vi "write wf.vi"() -> ()   [LabVIEW 2013]
uses:
  <vilib>/addons/database/Connection.llb/DB Tools Open Connec (Path).vi
  <vilib>/measure/NI_MABase.lvlib
  <vilib>/addons/database/NI_Database_API.lvlib
panel:
  out "error out":errorcluster
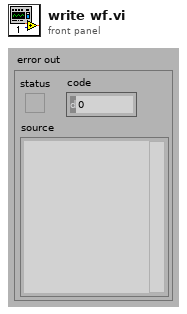
[diagram p1: front panel]
types:
  T1 = enum16{"Sine Wave", "Triangle Wave", "Square Wave", "Sawtooth Wave"}
  T2 = typedef "NI_Database_API.lvlib/Conn ObjectReference.ctl" = refnum<k1>
  T3 = cluster{"table":string, "signal out":waveform(dbl)}
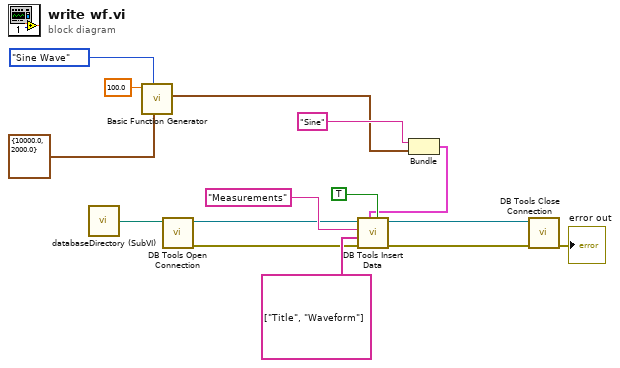
[diagram p0: block diagram]
diagram:
  n1 = call "databaseDirectory (SubVI).vi"() -> ("Application Directory"=w6:path)  [unwired: 1 in]
  n2 = call <vilib>:"Basic Function Generator.vi"("sampling info"=cluster{"Fs":dbl, "#s":dbl} {"Fs"=10000.0, "#s"=2000.0}, "signal type"=T1."Sine Wave", "frequency"=100.0) -> ("signal out"=w1:waveform(dbl))  [unwired: 6 in, 2 out]
  n3 = call-poly <vilib>:"DB Tools Open Connection.vi"("connection information"=w6) -> ("error out"=w5:errorcluster, "connection reference"=w4:T2)  [unwired: 7 in]
  n4 = Bundle("table"="Sine", "signal out"=w1) -> (w3:T3)  [unwired: 1 in]
  n5 = call <vilib>:"DB Tools Insert Data.vi"("create table? (F)"=TRUE ("create table? (f)"), "data"=w3, "error in (no error)"=w5, "columns"=string[] ["Title", "Waveform"], "table"="Measurements", "connection reference"=w4) -> ("error out"=w8:errorcluster, "connection reference out"=w9:T2)  [unwired: 4 in]
  n6 = call <vilib>:"DB Tools Close Connection.vi"("error in (no error)"=w8, "connection reference"=w9) -> ("error out"=→"error out":errorcluster)  [unwired: 5 in]
